vi "Get Command Line Arguments.vi"(4 "error in (no error)":errorcluster) -> (0 "error out":errorcluster, 2 "Values":string[](array[string]), 3 "Labels":string[](array[string]))   [LabVIEW 2015, in "Command Line Operations.lvlib"]
uses:
  Command Line Operations.lvlib
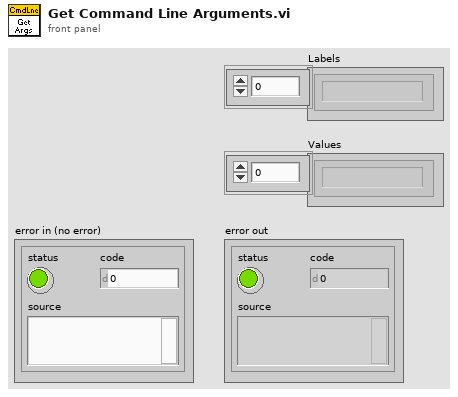
[diagram p1: front panel]
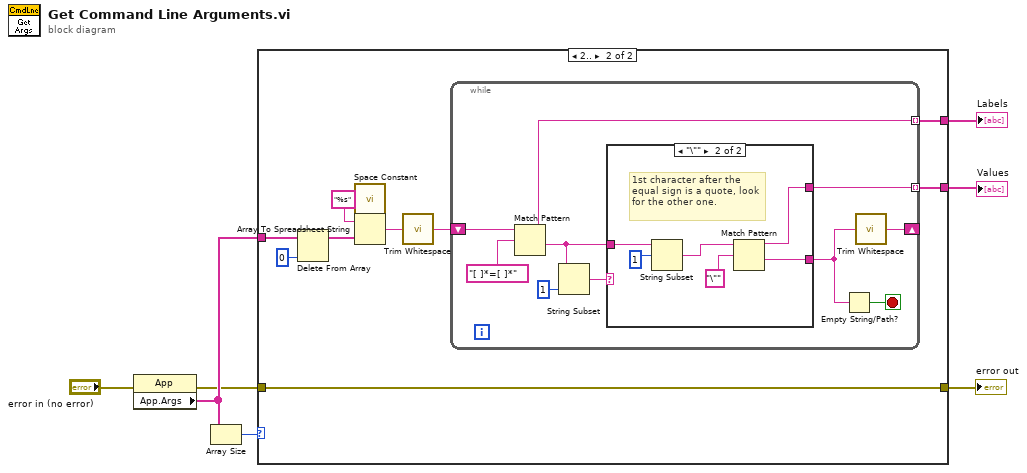
[diagram p0: block diagram]
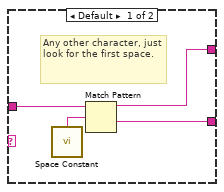
[diagram p3: hidden frame]
diagram:
  n1 = property class="App"(error in="error in (no error)") -> (error out=w3:errorcluster, "App.Args"=w4:string[])  [unwired: 1 in, 1 out]
  n2 = Array Size(array=w4) -> (size(s)=w2:i32)
  n3 = case shown="2.." w2 {
    tunnel: w3 -> [w8 w16]
    tunnel: w4 -> [_ w18]
    tunnel: [w8 w16] -> w5
    tunnel: [_ w10] -> w6
    tunnel: [_ w9] -> w7
    frame Default {
    }
    frame 2.. {
      n4 = Delete From Array(array=w18, index=0) -> (array with subset deleted=w15:string[])  [unwired: 1 in, 1 out]
      n5 = call <vilib>:"Space Constant.vi"() -> ("String"=w13:string)
      n6 = Array To Spreadsheet String(delimiter (Tab)=w13, array=w15, 3:"%s" ("format string")) -> (spreadsheet string=w12:string)
      n7 = call <vilib>:"Trim Whitespace.vi"("string"=w12) -> ("trimmed string"=w11:string)  [unwired: 1 in]
      n8 = while {
        shift-right: [w20] -> _
        shift-left: w11 -> [w28]
        tunnel: [w21] -> w10 mode=indexing
        tunnel: [w19] -> w9 mode=indexing
        stop <- w23 stop-if-true
        n9 = Match Pattern(string=w28, regular expression="[ ]*=[ ]*") -> (before substring=w21:string, after substring=w24:string)  [unwired: 1 in, 2 out]
        n10 = String Subset(string=w24, length (rest)=1 ("length (rest)")) -> (substring=w25:string)  [unwired: 1 in]
        n11 = case shown="\"\\\"\"" w25 {
          tunnel: w24 -> [w32 w37]
          tunnel: [w30 w34] -> w22
          tunnel: [w29 w33] -> w19
          frame Default {
            # "Any other character, just look for the first space."
            n12 = call <vilib>:"Space Constant.vi"() -> ("String"=w31:string)
            n13 = Match Pattern(string=w32, regular expression=w31) -> (before substring=w29:string, after substring=w30:string)  [unwired: 1 in, 2 out]
          }
          frame "\"" {
            # "1st character after the equal sign is a quote, look for the other one."
            n14 = String Subset(string=w37, offset (0)=1) -> (substring=w38:string)  [unwired: 1 in]
            n15 = Match Pattern(string=w38, regular expression="\"") -> (before substring=w33:string, after substring=w34:string)  [unwired: 1 in, 2 out]
          }
        }
        n16 = Empty String/Path?(string/path=w22) -> (empty?=w23:bool)
        n17 = call <vilib>:"Trim Whitespace.vi"("string"=w22) -> ("trimmed string"=w20:string)  [unwired: 1 in]
      }
    }
  }
  "Values" <- w7
  "Labels" <- w6
  "error out" <- w5
